vi "DAQ_DI.vi"(6 "Slot":T1, 8 "error in":errorcluster, 10 "CH":string, 11 "DAQConfig":refnum<vi>) -> (0 "error out":errorcluster, 3 "Status":bool)   [LabVIEW 2013]
uses:
  Controls/DAQConfig.ctl
  SystemCode/SysControl/Slot.ctl
  <vilib>/DAQmx/read.llb/DAQmx Read (Digital Bool 1Line 1Point).vi
  <vilib>/DAQmx/create/channels.llb/DAQmx Create Channel (DI-Digital Input).vi
  <vilib>/DAQmx/miscellaneous.llb/DAQmx Fill In Error Info.vi
panel:
  out "lines":tag caption="线"
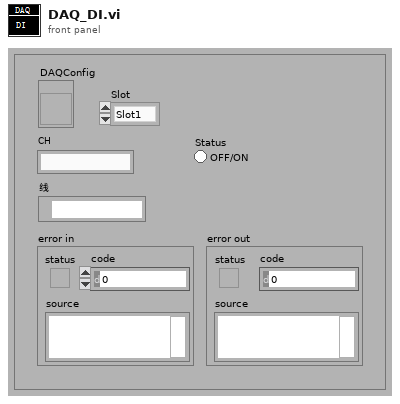
[diagram p1: front panel]
types:
  T1 = typedef "Slot.ctl" = enum16{"Slot1", "Slot2", "Slot3", "Slot4"}
  T2 = typedef "DAQConfig.ctl" = cluster{"DIO":string[][], "AO":string[][], "AI":string[][]}
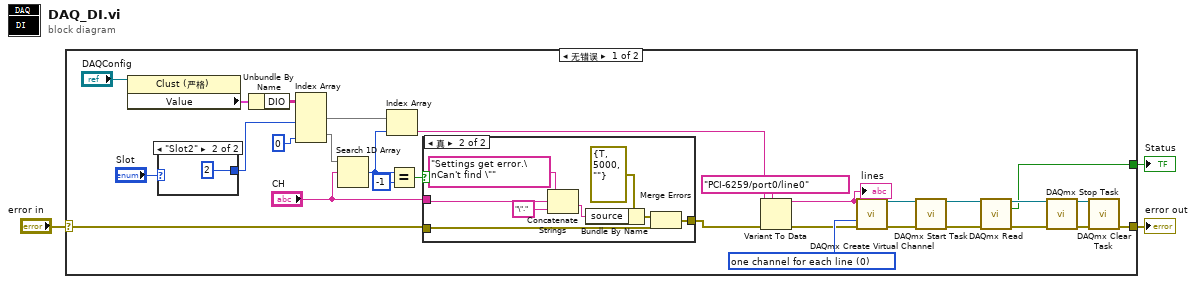
[diagram p0: block diagram]
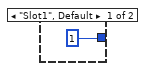
[diagram p2: hidden frame]
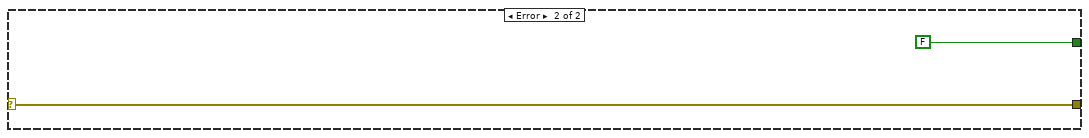
[diagram p4: hidden frame]
diagram:
  n1 = case shown="无错误" "error in" {
    selector: "error in" -> [w10 w45]
    tunnel: [w32 w45] -> w3
    tunnel: [w22 FALSE ("Boolean")] -> w1
    frame No Error {
      w23 = 0 items=["one channel for each line", "one channel for all lines"] ("line grouping")
      n2 = property class="Clust (严格)"(reference="DAQConfig") -> ("Value"=w18:T2)  [unwired: 1 in, 2 out]
      n3 = case shown="\"Slot2\"" "Slot" {
        tunnel: [1 ("索引 (行)") 2 ("索引 (行)")] -> w4
        frame "Slot1", Default {
        }
        frame "Slot2" {
        }
      }
      n4 = Unbundle By Name(w18) -> ("DIO"=w12:string[][])
      n5 = Index Array(array=w12, index (col) #1=w4, index (col) #2=0 ("索引 (列)")) -> (element #1=w7:string[], element #2=w8:string[])  [unwired: 2 in]
      n6 = Search 1D Array(1D array=w8, element="CH") -> (index of element=w14:i32)  [unwired: 1 in]
      n7 = Index Array(array=w7, index=w14) -> (element=w9:string)
      n8 = Equal?(x=w14, y=-1) -> (x = y?=w16:bool)
      n9 = case shown="真" w16 {
        tunnel: "CH" -> [_ w39]
        tunnel: w10 -> [w35 w37]
        tunnel: [w35 w36] -> w11
        frame False {
        }
        frame True {
          n10 = Concatenate Strings("Settings get error.\nCan't find \"" ("message"), w39, "\"." ("string")) -> (w42:string)
          n11 = Bundle By Name(cluster=errorcluster {"status"=TRUE, "code"=5000, "source"=""} ("error in 1 (no error)"), "source"=w42) -> (w41:errorcluster)
          n12 = Merge Errors(w41, w37) -> (w36:errorcluster)
        }
      }
      n13 = Variant To Data(error in=w11, type=tag "PCI-6259/port0/line0" ("lines"), Variant=w9) -> (data=w20:tag, error out=w19:errorcluster)
      "lines" <- w20
      n14 = call-poly <vilib>:"DAQmx Create Virtual Channel.vi"("lines"=w20, "line grouping"=w23, "error in"=w19) -> ("task out"=w31:refnum<k21>, "error out"=w30:errorcluster)  [unwired: 11 in]
      n15 = call <vilib>:"DAQmx Start Task.vi"("task/channels in"=w31, "error in"=w30) -> ("task out"=w29:refnum<k21>, "error out"=w28:errorcluster)  [unwired: 12 in]
      n16 = call-poly <vilib>:"DAQmx Read.vi"("task/channels in"=w29, "error in"=w28) -> ("task out"=w25:refnum<k21>, "data"=w22:bool, "error out"=w24:errorcluster)  [unwired: 11 in]
      n17 = call <vilib>:"DAQmx Stop Task.vi"("task/channels in"=w25, "error in"=w24) -> ("task out"=w27:refnum<k21>, "error out"=w26:errorcluster)  [unwired: 12 in]
      n18 = call <vilib>:"DAQmx Clear Task.vi"("task in"=w27, "error in"=w26) -> ("error out"=w32:errorcluster)  [unwired: 13 in]
    }
    frame Error {
    }
  }
  "error out" <- w3
  "Status" <- w1
